vi "Efficiency.vi"(8 "Maximum Power":dbl, 10 "Irradiance":dbl, 11 "Area":dbl) -> (3 "Efficiency":dbl)   [LabVIEW 2016]
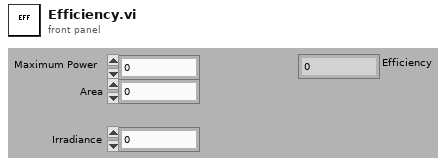
[diagram p1: front panel]
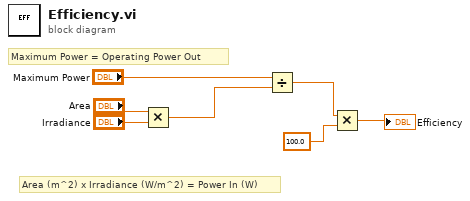
[diagram p0: block diagram]
diagram:
  # "Area (m^2) x Irradiance (W/m^2) = Power In (W)"
  # "Maximum Power = Operating Power Out"
  n1 = Multiply(x="Area", y="Irradiance") -> (x*y=w5:dbl)
  n2 = Divide(x="Maximum Power", y=w5) -> (x/y=w2:dbl)
  n3 = Multiply(x=w2, y=100.0) -> (x*y=→"Efficiency":dbl)
